vi "FGV Trigger.vi"(6 "Aktion":T3, 9 "Trigger setzen":bool, 11 "Triggerereignis":T1 {"Trigger verwenden" items=["Deaktiviert", "Aktiviert"]}) -> (0 "Trigger Eingang":bool, 1 "Trigger gesetzt?":bool, 2 "Trigger verwenden":bool, 3 "Triggerereignis neu":T1 {"Trigger verwenden" items=["Deaktiviert", "Aktiviert"]})   [LabVIEW 2020, in "LogKonfig.lvlib"]
uses:
  LogKonfig.lvlib
  Aktionen Trigger.ctl
  Element Triggerereignisse.ctl
  Auswahlfeld aktiviert-deaktiviert.ctl
  cRIO/PC/Kommunikation mit cRIO.lvlib
panel:
  out "Puffergröße":sgl
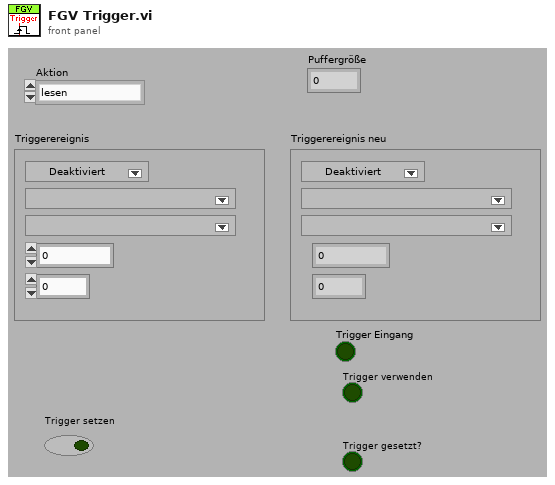
[diagram p1: front panel]
types:
  T1 = typedef "LogKonfig.lvlib/Element Triggerereignisse.ctl" = cluster{"Trigger verwenden":T2, "Messwert":u16, "kl./gr.":u16, "Wert":sgl, "Puffergröße":sgl}
  T2 = typedef "LogKonfig.lvlib/Auswahlfeld aktiviert-deaktiviert.ctl" = u16
  T3 = typedef "LogKonfig.lvlib/Aktionen Trigger.ctl" = enum16{"lesen", "ALLE schreiben", "Trigger prüfen", "Trigger rücksetzen"}
  T4 = typedef "Verwaltung - cRIO.lvlib/Digital Eingaenge 0-15.ctl" = cluster{"I0: N2 Nachf. FT-IR voll":bool, "I1: N2 Nachf. Vorrat leer":bool, "I2: (Klimaanlage eingeschaltet)":bool, "I3: (Klimaanlage Störung)":bool, "I4: Trigger Eingang (Messdaten sp.)":bool, "I5: Reserve":bool, "I6: Reserve":bool, "I7: Reserve":bool, "I8: Druckschalter Versorgung ok":bool, "I9: Reserve":bool, "I10: Reserve":bool, "I11: Reserve":bool, "I12: Drucksch. N2 Versorgung":bool, "I13: Reserve":bool, "I14: Drucksch. N2 Optikbox":bool, "I15: (Füllstand Kondensatbehälter)":bool}
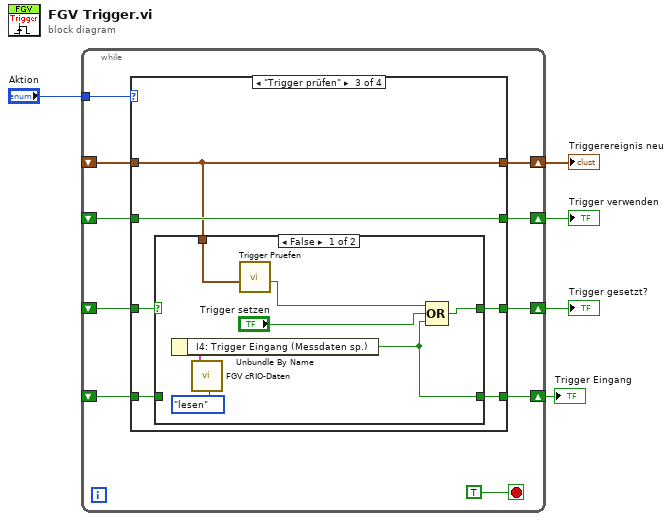
[diagram p0: block diagram]
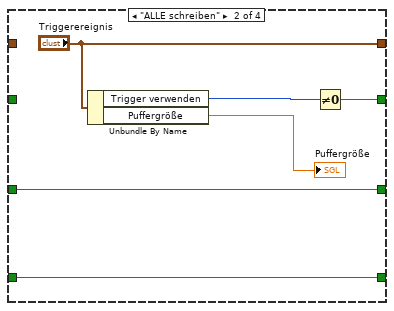
[diagram p3: hidden frame]
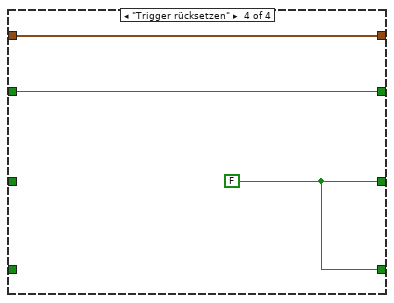
[diagram p5: hidden frame]
diagram:
  n1 = while {
    tunnel: "Aktion" -> [w14]
    shift-right: [w13] -> w4
    shift-left: _ -> [w12]
    shift-right: [w11] -> w3
    shift-left: _ -> [w10]
    shift-right: [w9] -> w2
    shift-left: _ -> [w8]
    shift-right: [w7] -> w1
    shift-left: _ -> [w6]
    stop <- TRUE stop-if-true
    n2 = case shown="\"Trigger prüfen\"" w14 {
      tunnel: [w19 "Triggerereignis" w29 w43] -> w13
      tunnel: w12 -> [w19 _ w29 w43]
      tunnel: [w18 w23 w31 w42] -> w11
      tunnel: w10 -> [w18 _ w31 w42]
      tunnel: [w17 w22 w30 w41] -> w9
      tunnel: w8 -> [w17 w22 w28 _]
      tunnel: [w16 w20 w27 w41] -> w7
      tunnel: w6 -> [w16 w20 w26 _]
      frame "lesen", Default {
      }
      frame "ALLE schreiben" {
        n3 = Unbundle By Name("Triggerereignis") -> ("Trigger verwenden"=w24:T2, "Puffergröße"=→"Puffergröße":sgl)
        n4 = Not Equal To 0?(x=w24) -> (x != 0?=w23:bool)
      }
      frame "Trigger prüfen" {
        n5 = case shown="False" w28 {
          selector: w28 -> [_ w40]
          tunnel: [w35 w40] -> w30
          tunnel: w29 -> [w38 _]
          tunnel: [w32 w39] -> w27
          tunnel: w26 -> [_ w39]
          frame False {
            n6 = call "FGV cRIO-Daten.vi"("Aktion"=enum16{"lesen", "schreiben"}."lesen") -> ("DI"=w33:T4)  [unwired: 9 in, 9 out]
            n7 = Unbundle By Name(w33) -> ("I4: Trigger Eingang (Messdaten sp.)"=w32:bool)
            n8 = call "Trigger Pruefen.vi"("Triggerereignis"=w38) -> ("Trigger"=w37:bool)  [unwired: 10 in]
            n9 = Compound Arithmetic op=OR(w37, "Trigger setzen", w32) -> (w35:bool)
          }
          frame True {
          }
        }
      }
      frame "Trigger rücksetzen" {
        w41 = FALSE
      }
    }
  }
  "Triggerereignis neu" <- w4
  "Trigger verwenden" <- w3
  "Trigger gesetzt?" <- w2
  "Trigger Eingang" <- w1
